vi "Constants.vi"() -> ()   [LabVIEW 2011, in "KinectOne.lvlib"]
uses:
  KinectOne.lvlib
panel:
  in  "InferredZPositionClamp":sgl=0.1
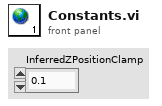
[diagram p1: front panel]
diagram:
